vi "Create Temporary Template Directory.vi"(9 "Kernel LVLib Dir":path=path "C:/LQWidgets", 11 "Template LVLib":refnum<vi>) -> (2 "Temporary Template Root Dir":path, 3 "Template LVLib Dup":refnum<vi>)   [LabVIEW 2013]
uses:
  <vilib>/Utility/sysdir.llb/System Directory Type.ctl
  <vilib>/Utility/traverseref.llb/TRef TravTarget.ctl
  <vilib>/Utility/traverseref.llb/VI Scripting - Traverse.lvlib
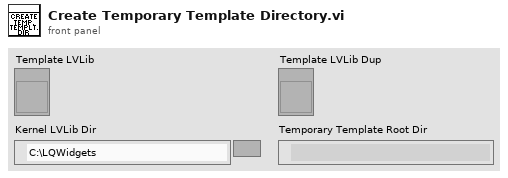
[diagram p1: front panel]
types:
  T1 = typedef "System Directory Type.ctl" = i32
  T2 = typedef "TRef TravTarget.ctl" = enum16{"FP", "BD", "Other"}
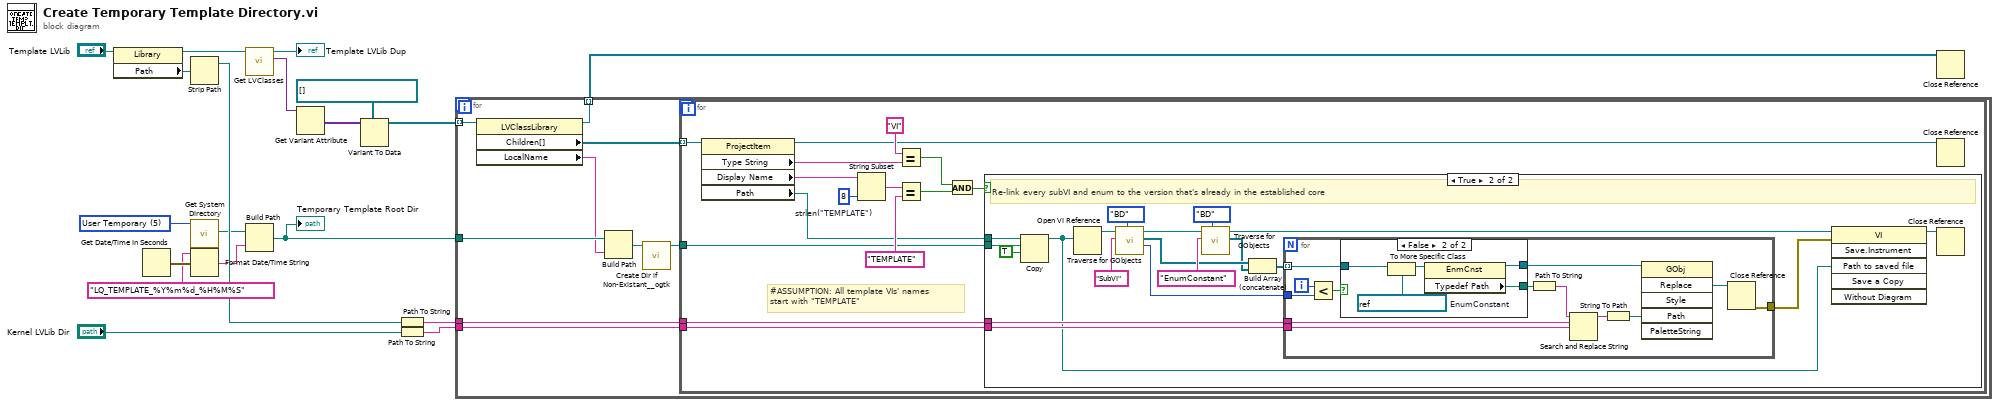
[diagram p0: block diagram]
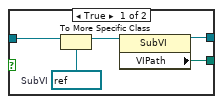
[diagram p3: hidden frame]
diagram:
  w6 = T1 5 items=["User Home"=0, "User Desktop"=1, "User Documents"=2, "User Application Data"=3, "User Preferences"=4, "User Temporary"=5, "Public Documents"=6, "Public Application Data"=7, "Public Preferences"=8, "Public Cache"=13, "System Core Libraries"=9, "System Installed Libraries"=10, "Application Files"=11, "Boot Volume Root"=12] ("system directory type")
  n1 = property class="Library"(reference="Template LVLib") -> (reference out=w9:refnum<vi>, "Path"=w11:path)  [unwired: 1 in, 1 out]
  n2 = Get Date/Time In Seconds() -> (seconds since 1Jan1904=w3:timestamp)
  n3 = Strip Path(path=w11) -> (stripped path=w14:path)  [unwired: 1 out]
  n4 = call <vilib>:"Get System Directory.vi"("system directory type"=w6) -> ("system directory"=w5:path)  [unwired: 10 in]
  n5 = Format Date/Time String(time format string (%c)="LQ_TEMPLATE_%Y%m%d_%H%M%S", seconds (now)=w3) -> (date/time string=w4:string)  [unwired: 1 in]
  n6 = call "Get LVClasses.vi"("LVLib"=w9) -> ("Class Ref Map"=w19:variant, "LVLib Dup"=→"Template LVLib Dup":refnum<vi>)  [unwired: 9 in]
  n7 = Build Path(base path=w5, name or relative path=w4) -> (appended path=w1:path)
  "Temporary Template Root Dir" <- w1
  n8 = Get Variant Attribute(Variant=w19) -> (values=w18:variant[])  [unwired: 3 in, 3 out]
  n9 = Variant To Data(type=refnum<vi>[] [], Variant=w18) -> (data=w16:refnum<vi>[])  [unwired: 1 in, 1 out]
  n10 = Path To String(path=w14) -> (string=w13:string)
  n11 = Path To String(path="Kernel LVLib Dir") -> (string=w12:string)
  n12 = for {
    tunnel: w16 -> [w28] mode=indexing
    tunnel: w1 -> [w26]
    tunnel: w13 -> [w22]
    tunnel: w12 -> [w21]
    tunnel: [w20] -> w7 mode=indexing
    n13 = property class="LVClassLibrary"(reference=w28) -> (reference out=w20:refnum<vi>, "Children[]"=w27:refnum<vi>[], "LocalName"=w25:string)  [unwired: 1 in, 1 out]
    n14 = Build Path(base path=w26, name or relative path=w25) -> (appended path=w24:path)
    n15 = call <userlib>:"Create Dir if Non-Existant__ogtk.vi"("Directory Path"=w24) -> ("dup Directory Path"=w23:path)  [unwired: 8 in, 2 out]
    n16 = for {
      tunnel: w27 -> [w43] mode=indexing
      tunnel: w23 -> [w33]
      tunnel: w22 -> [w32]
      tunnel: w21 -> [w31]
      w42 = 8  # strlen("TEMPLATE")
      # "#ASSUMPTION: All template VIs' names\nstart with \"TEMPLATE\""
      n17 = property class="ProjectItem"(reference=w43) -> (reference out=w34:refnum<vi>, "Type String"=w39:string, "Display Name"=w30:string, "Path"=w29:path)  [unwired: 1 in, 1 out]
      n18 = String Subset(string=w30, length (rest)=w42) -> (substring=w41:string)  [unwired: 1 in]
      n19 = Equal?(x="VI" ("y"), y=w39) -> (x = y?=w36:bool)
      n20 = Equal?(x=w41, y="TEMPLATE") -> (x = y?=w37:bool)
      n21 = And(x=w36, y=w37) -> (x .and. y?=w35:bool)
      n22 = case shown="True" w35 {
        tunnel: w29 -> [_ w62]
        tunnel: w33 -> [_ w61]
        tunnel: w32 -> [_ w56]
        tunnel: w31 -> [_ w55]
        frame False {
        }
        frame True {
          # "Re-link every subVI and enum to the version that's already in the established core"
          n23 = Copy(9:TRUE ("overwrite (F)"), 10:w61, 11:w62) -> (3:w53:path)  [unwired: 2 in, 2 out]
          n24 = Open VI Reference(vi path=w53) -> (vi reference=w57:refnum<vi>)  [unwired: 5 in, 1 out]
          n25 = call <vilib>:"Traverse for GObjects.vi"("Traverse Target"=TRef_TravTarget."BD", "Class Name"="SubVI", "VI Refnum"=w57) -> ("# of Refs"=w51:i32, "References"=w46:refnum<vi>[], "dup VI Refnum"=w48:refnum<vi>)  [unwired: 5 in, 1 out]
          n26 = call <vilib>:"Traverse for GObjects.vi"("Traverse Target"=TRef_TravTarget."BD", "Class Name"="EnumConstant", "VI Refnum"=w48) -> ("References"=w44:refnum<vi>[], "dup VI Refnum"=w47:refnum<vi>)  [unwired: 5 in, 2 out]
          n27 = Build Array (concatenate)(w46, w44) -> (w45:refnum<vi>[])
          n28 = for {
            tunnel: w45 -> [w75] mode=indexing
            tunnel: w56 -> [w71]
            tunnel: w55 -> [w70]
            tunnel: [w66] -> w54
            tunnel: w51 -> [w64]
            i -> [w65]
            n29 = Less?(x=w65, y=w64) -> (x < y?=w63:bool)
            n30 = case shown="False" w63 {
              tunnel: w75 -> [w80 w85]
              tunnel: [w77 w82] -> w74
              tunnel: [w76 w81] -> w73
              frame True {
                w79 = refnum<vi> refnum  # SubVI
                n31 = To More Specific Class(target class=w79, reference=w80) -> (specific class reference=w78:refnum<vi>)  [unwired: 1 in, 1 out]
                n32 = property class="SubVI"(reference=w78) -> (reference out=w77:refnum<vi>, "VIPath"=w76:path)  [unwired: 1 in, 1 out]
              }
              frame False {
                w84 = refnum<vi> refnum  # EnumConstant
                n33 = To More Specific Class(target class=w84, reference=w85) -> (specific class reference=w83:refnum<vi>)  [unwired: 1 in, 1 out]
                n34 = property class="EnmCnst"(reference=w83) -> (reference out=w82:refnum<vi>, "Typedef Path"=w81:path)  [unwired: 1 in, 1 out]
              }
            }
            n35 = Path To String(path=w73) -> (string=w72:string)
            n36 = Search and Replace String(input string=w72, search string=w71, replace string=w70) -> (result string=w69:string)  [unwired: 5 in, 3 out]
            n37 = String To Path(string=w69) -> (path=w68:path)
            n38 = invoke class="GObj" method="Replace"(reference=w74, "Path"=w68) -> ("Replace"=w67:refnum<vi>)  [unwired: 4 in, 5 out]
            n39 = Close Reference(reference=w67) -> (error out=w66:errorcluster)  [unwired: 1 in]
          }
          n40 = invoke class="VI" method="Save.Instrument"(reference=w47, error in=w54, "Path to saved file"=w53) -> (reference out=w52:refnum<vi>)  [unwired: 3 in, 5 out]
          n41 = Close Reference(reference=w52) -> ()  [unwired: 1 in, 1 out]
        }
      }
      n42 = Close Reference(reference=w34) -> ()  [unwired: 1 in, 1 out]
    }
  }
  n43 = Close Reference(reference=w7) -> ()  [unwired: 1 in, 1 out]
